vi "Wait Valve Actuate.vi"(1 "error in":errorcluster) -> (0 "error out":errorcluster)   [LabVIEW 2018]
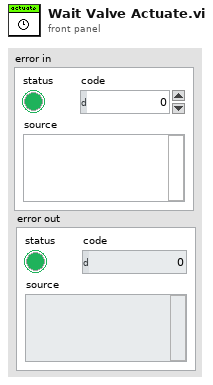
[diagram p1: front panel]
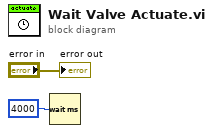
[diagram p0: block diagram]
diagram:
  n1 = Wait (ms)(milliseconds to wait=u32 4000) -> ()  [unwired: 1 out]
  "error out" <- "error in"
